vi "Register Dynamic Events.vi"(8 "error in (no error)":errorcluster, 11 "ListboxEventHandler In":refnum<class "ListboxEventHandler.lvclass">) -> (0 "error out":errorcluster, 3 "ListboxEventHandler Out":refnum<class "ListboxEventHandler.lvclass">)   [LabVIEW 2015, in "ActorEvents.lvlib" / "ListboxEventHandler.lvclass"]
uses:
  ListboxEventHandler.lvclass
  IEventHandler/IEventHandler.lvclass/IEventHandler.ctl
  <vilib>/event_ctls.llb/lveventtype.ctl
  ListboxEventHandler.lvclass/ListboxEventHandler.ctl
  IEventHandler/Read Registrations.vi
  IEventHandler/IEventHandler.lvclass
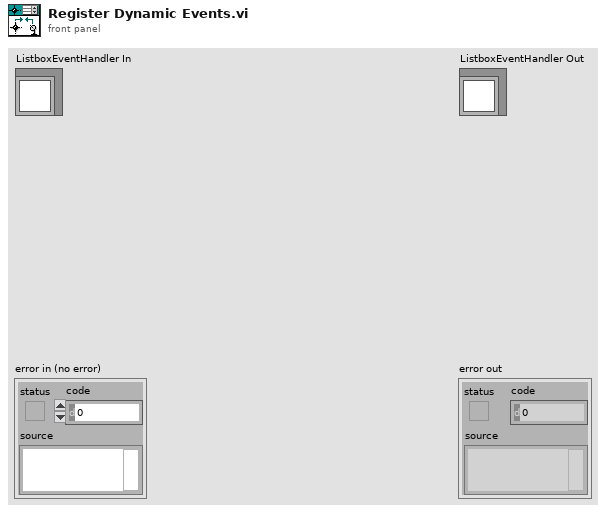
[diagram p1: front panel]
types:
  T1 = typedef "lveventtype.ctl" = enum32{"Null", "Timeout", "Annotation Menu Selection", "Annotation Menu Selection?", "App Instance Close", "App Instance Close?", "Autoscale Range Change", "Bookmark Info Change", "Cell Edit", "Cell Edit?", "Cursor Grab", "Cursor Grab?", "Cursor Menu Selection", "Cursor Menu Selection?", "Cursor Move", "Cursor Release", "Data Change", "Direction Change", "Display State Change", "Drag Ended", "Drag Enter", "Drag Leave", "Drag Over", "Drag Source Update", "Drag Starting", "Drag Starting?", "Drop", "Exec State Change", "Key Down", "Key Down?", "Key Repeat", "Key Repeat?", "Key Up", "Listbox Double Click", "Menu Activation?", "Menu Selection (App)", "Menu Selection? (App)", "Menu Selection (User)", "Mouse Down", "Mouse Down?", "Mouse Enter", "Mouse Leave", "Mouse Move", "Mouse Up", "Mouse Wheel", "NI Security User Change (App)", "Pane Size", "Panel Close", "Panel Close?", "Panel Resize", "Plot Attribute Change", "Scale Range Change", "Shortcut Menu Activation?", "Shortcut Menu Selection (App)", "Shortcut Menu Selection? (App)", "Shortcut Menu Selection (User)", "Tree Double Click", "Tree Drag", "Tree Drag?", "Tree Drop", "Tree Drop?", "Tree Item Close", "Tree Item Close?", "Tree Item Open", "Tree Item Open?", "User Event", "Value Change"}
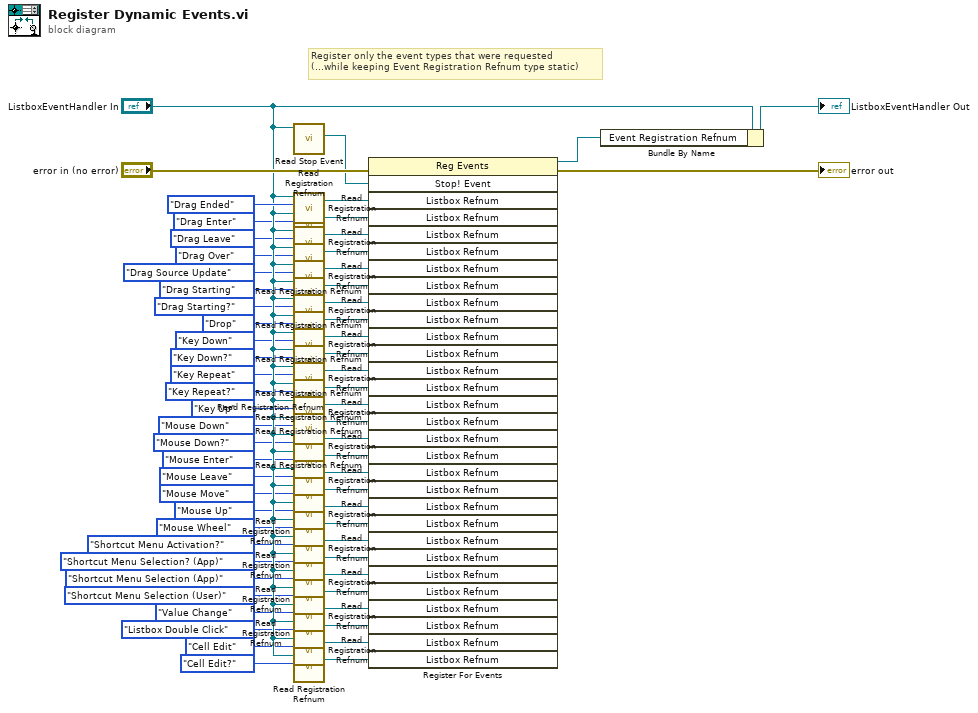
[diagram p0: block diagram]
diagram:
  # "Register only the event types that were requested\n(...while keeping Event Registration Refnum type static)"
  n1 = call "Read Stop Event.vi"("IEventHandler in"="ListboxEventHandler In") -> ("Stop! Event"=w61:refnum<user-event>)  [unwired: 10 in]
  n2 = call "Read Registration Refnum.vi"("Event Type"=lveventtype."Drag Ended", "ListboxEventHandler"="ListboxEventHandler In") -> ("Listbox Refnum"=w32:refnum<vi>)  [unwired: 5 in]
  n3 = call "Read Registration Refnum.vi"("Event Type"=lveventtype."Drag Enter", "ListboxEventHandler"="ListboxEventHandler In") -> ("Listbox Refnum"=w31:refnum<vi>)  [unwired: 5 in]
  n4 = call "Read Registration Refnum.vi"("Event Type"=lveventtype."Drag Leave", "ListboxEventHandler"="ListboxEventHandler In") -> ("Listbox Refnum"=w30:refnum<vi>)  [unwired: 5 in]
  n5 = call "Read Registration Refnum.vi"("Event Type"=lveventtype."Drag Over", "ListboxEventHandler"="ListboxEventHandler In") -> ("Listbox Refnum"=w29:refnum<vi>)  [unwired: 5 in]
  n6 = call "Read Registration Refnum.vi"("Event Type"=lveventtype."Drag Source Update", "ListboxEventHandler"="ListboxEventHandler In") -> ("Listbox Refnum"=w28:refnum<vi>)  [unwired: 5 in]
  n7 = call "Read Registration Refnum.vi"("Event Type"=lveventtype."Drag Starting", "ListboxEventHandler"="ListboxEventHandler In") -> ("Listbox Refnum"=w27:refnum<vi>)  [unwired: 5 in]
  n8 = call "Read Registration Refnum.vi"("Event Type"=lveventtype."Drag Starting?", "ListboxEventHandler"="ListboxEventHandler In") -> ("Listbox Refnum"=w26:refnum<vi>)  [unwired: 5 in]
  n9 = call "Read Registration Refnum.vi"("Event Type"=lveventtype."Drop", "ListboxEventHandler"="ListboxEventHandler In") -> ("Listbox Refnum"=w25:refnum<vi>)  [unwired: 5 in]
  n10 = call "Read Registration Refnum.vi"("Event Type"=lveventtype."Key Down", "ListboxEventHandler"="ListboxEventHandler In") -> ("Listbox Refnum"=w24:refnum<vi>)  [unwired: 5 in]
  n11 = call "Read Registration Refnum.vi"("Event Type"=lveventtype."Key Down?", "ListboxEventHandler"="ListboxEventHandler In") -> ("Listbox Refnum"=w23:refnum<vi>)  [unwired: 5 in]
  n12 = call "Read Registration Refnum.vi"("Event Type"=lveventtype."Key Repeat", "ListboxEventHandler"="ListboxEventHandler In") -> ("Listbox Refnum"=w22:refnum<vi>)  [unwired: 5 in]
  n13 = call "Read Registration Refnum.vi"("Event Type"=lveventtype."Key Repeat?", "ListboxEventHandler"="ListboxEventHandler In") -> ("Listbox Refnum"=w21:refnum<vi>)  [unwired: 5 in]
  n14 = call "Read Registration Refnum.vi"("Event Type"=lveventtype."Key Up", "ListboxEventHandler"="ListboxEventHandler In") -> ("Listbox Refnum"=w20:refnum<vi>)  [unwired: 5 in]
  n15 = call "Read Registration Refnum.vi"("Event Type"=lveventtype."Mouse Down", "ListboxEventHandler"="ListboxEventHandler In") -> ("Listbox Refnum"=w19:refnum<vi>)  [unwired: 5 in]
  n16 = call "Read Registration Refnum.vi"("Event Type"=lveventtype."Mouse Down?", "ListboxEventHandler"="ListboxEventHandler In") -> ("Listbox Refnum"=w18:refnum<vi>)  [unwired: 5 in]
  n17 = call "Read Registration Refnum.vi"("Event Type"=lveventtype."Mouse Enter", "ListboxEventHandler"="ListboxEventHandler In") -> ("Listbox Refnum"=w17:refnum<vi>)  [unwired: 5 in]
  n18 = call "Read Registration Refnum.vi"("Event Type"=lveventtype."Mouse Leave", "ListboxEventHandler"="ListboxEventHandler In") -> ("Listbox Refnum"=w16:refnum<vi>)  [unwired: 5 in]
  n19 = call "Read Registration Refnum.vi"("Event Type"=lveventtype."Mouse Move", "ListboxEventHandler"="ListboxEventHandler In") -> ("Listbox Refnum"=w15:refnum<vi>)  [unwired: 5 in]
  n20 = call "Read Registration Refnum.vi"("Event Type"=lveventtype."Mouse Up", "ListboxEventHandler"="ListboxEventHandler In") -> ("Listbox Refnum"=w14:refnum<vi>)  [unwired: 5 in]
  n21 = call "Read Registration Refnum.vi"("Event Type"=lveventtype."Mouse Wheel", "ListboxEventHandler"="ListboxEventHandler In") -> ("Listbox Refnum"=w13:refnum<vi>)  [unwired: 5 in]
  n22 = call "Read Registration Refnum.vi"("Event Type"=lveventtype."Shortcut Menu Activation?", "ListboxEventHandler"="ListboxEventHandler In") -> ("Listbox Refnum"=w12:refnum<vi>)  [unwired: 5 in]
  n23 = call "Read Registration Refnum.vi"("Event Type"=lveventtype."Shortcut Menu Selection? (App)", "ListboxEventHandler"="ListboxEventHandler In") -> ("Listbox Refnum"=w11:refnum<vi>)  [unwired: 5 in]
  n24 = call "Read Registration Refnum.vi"("Event Type"=lveventtype."Shortcut Menu Selection (App)", "ListboxEventHandler"="ListboxEventHandler In") -> ("Listbox Refnum"=w10:refnum<vi>)  [unwired: 5 in]
  n25 = call "Read Registration Refnum.vi"("Event Type"=lveventtype."Shortcut Menu Selection (User)", "ListboxEventHandler"="ListboxEventHandler In") -> ("Listbox Refnum"=w9:refnum<vi>)  [unwired: 5 in]
  n26 = call "Read Registration Refnum.vi"("Event Type"=lveventtype."Value Change", "ListboxEventHandler"="ListboxEventHandler In") -> ("Listbox Refnum"=w8:refnum<vi>)  [unwired: 5 in]
  n27 = call "Read Registration Refnum.vi"("Event Type"=lveventtype."Listbox Double Click", "ListboxEventHandler"="ListboxEventHandler In") -> ("Listbox Refnum"=w7:refnum<vi>)  [unwired: 5 in]
  n28 = call "Read Registration Refnum.vi"("Event Type"=lveventtype."Cell Edit", "ListboxEventHandler"="ListboxEventHandler In") -> ("Listbox Refnum"=w5:refnum<vi>)  [unwired: 5 in]
  n29 = call "Read Registration Refnum.vi"("Event Type"=lveventtype."Cell Edit?", "ListboxEventHandler"="ListboxEventHandler In") -> ("Listbox Refnum"=w2:refnum<vi>)  [unwired: 5 in]
  n30 = register-events(error in="error in (no error)", w61, w32, w31, w30, w29, w28, w27, w26, w25, w24, w23, w22, w21, w20, w19, w18, w17, w16, w15, w14, w13, w12, w11, w10, w9, w8, w7, w5, w2) -> (reference out=w1:refnum<event-registration>, error out=→"error out":errorcluster)  [unwired: 1 in]
  n31 = Bundle By Name(cluster="ListboxEventHandler In", "Event Registration Refnum"=w1) -> (→"ListboxEventHandler Out":refnum<class "ListboxEventHandler.lvclass">)
